vi "dvp Vi Set Flip Vertical State.vi"(10 "FlipVerticalState":i32, 11 "handle":u32) -> (3 "function return":u32(ring))   [LabVIEW 2018, in "LabViewDVPCamera.lvlib"]
doc: "LabviewDvp2Api dvpStatus dvpViSetFlipVerticalState(dvpHandle handle, BOOL FlipVerticalState);"
uses:
  LabViewDVPCamera.lvlib
  LabViewDVPCamera/LabViewDVPCamera.dll
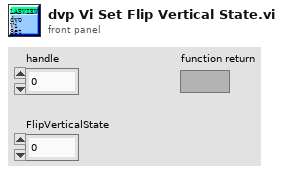
[diagram p1: front panel]
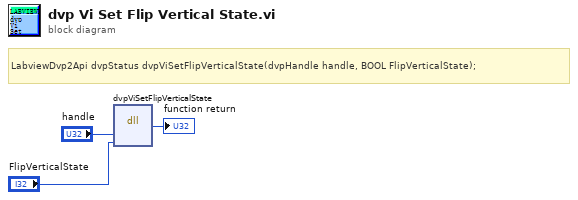
[diagram p0: block diagram]
diagram:
  # "LabviewDvp2Api dvpStatus dvpViSetFlipVerticalState(dvpHandle handle, BOOL FlipVerticalState);"
  n1 = dll-call lib="C:/Program Files (x86)/DVP2 Labview cn 64/Sample/LabViewDVPCamera/LabViewDVPCamera.*" fn="dvpViSetFlipVerticalState"("handle"="handle", "FlipVerticalState"="FlipVerticalState") -> (→"function return":u32)  [unwired: 5 in, 2 out]
